vi "Flatness_ON-OFF.vi"(0 "Session In":refnum<visa-resource-name>="TCPIP0::169.254.70.100::inst0::INSTR", 2 "RO(T)":bool, 11 "error in":errorcluster {"code" format="%.0x"}, 12 "CORR ON(T)":bool) -> (3 "success":bool, 4 "Session Out":refnum<visa-resource-name>="TCPIP0::169.254.70.100::inst0::INSTR", 15 "error out":errorcluster {"code" format="%.0x"})   [LabVIEW 2018]
doc: "Launches the Instrument I/O Assistant, which you can use to communicate with message-based instruments and graphically parse the response. For example you can communicate with an instrument that uses a serial, Ethernet, or GPIB interface."
panel:
  in  "Timeout":u32=3000
  out "corr on(t)":bool
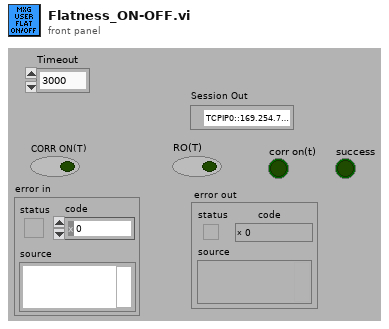
[diagram p1: front panel]
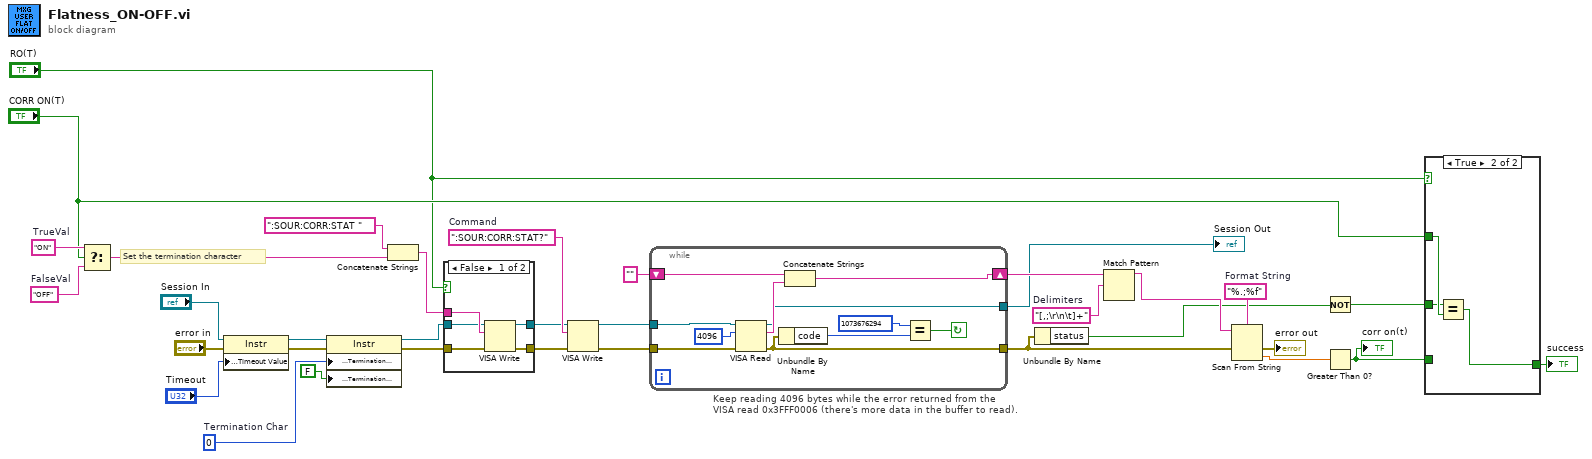
[diagram p0: block diagram]
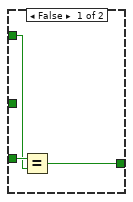
[diagram p2: hidden frame]
diagram:
  w12 = "[,;\r\n\t]+"  # Delimiters
  w14 = "%.;%f"  # Format String
  w17 = ":SOUR:CORR:STAT?"  # Command
  w27 = u8 0  # Termination Char
  w32 = "OFF"  # FalseVal
  w33 = "ON"  # TrueVal
  # "Keep reading 4096 bytes while the error returned from the\nVISA read 0x3FFF0006 (there's more data in the buffer to read)."
  # "Set the termination character"
  n1 = Select(t=w33, s="CORR ON(T)", f=w32) -> (s? t:f=w24:string)
  n2 = property class="Instr"(reference="Session In", error in="error in", "General Settings:Timeout Value"="Timeout") -> (reference out=w26:refnum<visa-resource-name>, error out=w29:errorcluster)
  n3 = property class="Instr"(reference=w26, error in=w29, "Message Based Settings:Termination Character"=w27, "Message Based Settings:Termination Character Enable"=FALSE ("enable")) -> (reference out=w11:refnum<visa-resource-name>, error out=w28:errorcluster)
  n4 = Concatenate Strings(":SOUR:CORR:STAT " ("staticText"), w24) -> (w21:string)
  n5 = case shown="False" "RO(T)" {
    tunnel: w28 -> [w39 w41]
    tunnel: [w38 w41] -> w22
    tunnel: w21 -> [w37 _]
    tunnel: w11 -> [w36 w40]
    tunnel: [w35 w40] -> w9
    frame False {
      n6 = VISA Write(VISA resource name=w36, write buffer=w37, error in (no error)=w39) -> (VISA resource name out=w35:refnum<visa-resource-name>, error out=w38:errorcluster)  [unwired: 1 out]
    }
    frame True {
    }
  }
  n7 = VISA Write(VISA resource name=w9, write buffer=w17, error in (no error)=w22) -> (VISA resource name out=w20:refnum<visa-resource-name>, error out=w19:errorcluster)  [unwired: 1 out]
  n8 = while {
    tunnel: w20 -> [w49]
    shift-right: [w43] -> w16
    shift-left: "" -> [w48]
    tunnel: w19 -> [w46]
    tunnel: [w45] -> w5
    tunnel: [w42] -> w1
    stop <- w44 continue-if-true
    n9 = VISA Read(VISA resource name=w49, byte count=u32 4096 ("byte count (0)"), error in (no error)=w46) -> (VISA resource name out=w42:refnum<visa-resource-name>, read buffer=w47:string, error out=w45:errorcluster)  [unwired: 1 out]
    n10 = Unbundle By Name(w45) -> ("code"=w51:i32)
    n11 = Concatenate Strings(w48, w47) -> (w43:string)
    n12 = Equal?(x=1073676294, y=w51) -> (x = y?=w44:bool)
  }
  "Session Out" <- w1
  n13 = Unbundle By Name(w5) -> ("status"=w4:bool)
  n14 = Match Pattern(string=w16, regular expression=w12) -> (before substring=w15:string)  [unwired: 1 in, 3 out]
  n15 = Scan From String(format string=w14, input string=w15, error in=w5) -> (error out=→"error out":errorcluster, output 1=w10:dbl)  [unwired: 2 in, 2 out]
  n16 = Not(x=w4) -> (.not. x?=w2:bool)
  n17 = Greater Than 0?(x=w10) -> (x > 0?=w8:bool)
  "corr on(t)" <- w8
  n18 = case shown="True" "RO(T)" {
    tunnel: w8 -> [w55 _]
    tunnel: "CORR ON(T)" -> [w54 w58]
    tunnel: [w53 w57] -> w6
    tunnel: w2 -> [_ w56]
    frame False {
      n19 = Equal?(x=w55, y=w54) -> (x = y?=w53:bool)
    }
    frame True {
      n20 = Equal?(x=w56, y=w58) -> (x = y?=w57:bool)
    }
  }
  "success" <- w6
